vi "PTP.vi"() -> ()   [LabVIEW 2019]
panel:
  in  "Vision&Robot":T1(array[cluster])=[{"VisionPoint"={"X"=7.711431, "Y"=-4.299606}, "RobotPoint"={"X"=148.386, "Y"=76.831, "U"=0.0}}, {"VisionPoint"={"X"=213.378555, "Y"=-5.1972}, "RobotPoint"={"X"=351.958, "Y"=82.394, "U"=0.0}}, {"VisionPoint"={"X"=7.918081, "Y"=146.750031}, "RobotPoint"={"X"=152.021, "Y"=-78.481, "U"=0.0}}, {"VisionPoint"={"X"=220.545044, "Y"=146.174713}, "RobotPoint"={"X"=356.701, "Y"=-69.132, "U"=0.0}}, {"VisionPoint"={"X"=0.0, "Y"=0.0}, "RobotPoint"={"X"=0.0, "Y"=0.0, "U"=0.0}}, {"VisionPoint"={"X"=0.0, "Y"=0.0}, "RobotPoint"={"X"=0.0, "Y"=0.0, "U"=0.0}}, {"VisionPoint"={"X"=0.0, "Y"=0.0}, "RobotPoint"={"X"=0.0, "Y"=0.0, "U"=0.0}}]
  out "RobotOut(B )":cluster{"RX":dbl, "RY":dbl}
  in  "InputRobot(B)":T2
  in  "ImgPoint":T2
  in  "ImgPoint":cluster{"PTX1":dbl, "PTY1":dbl}
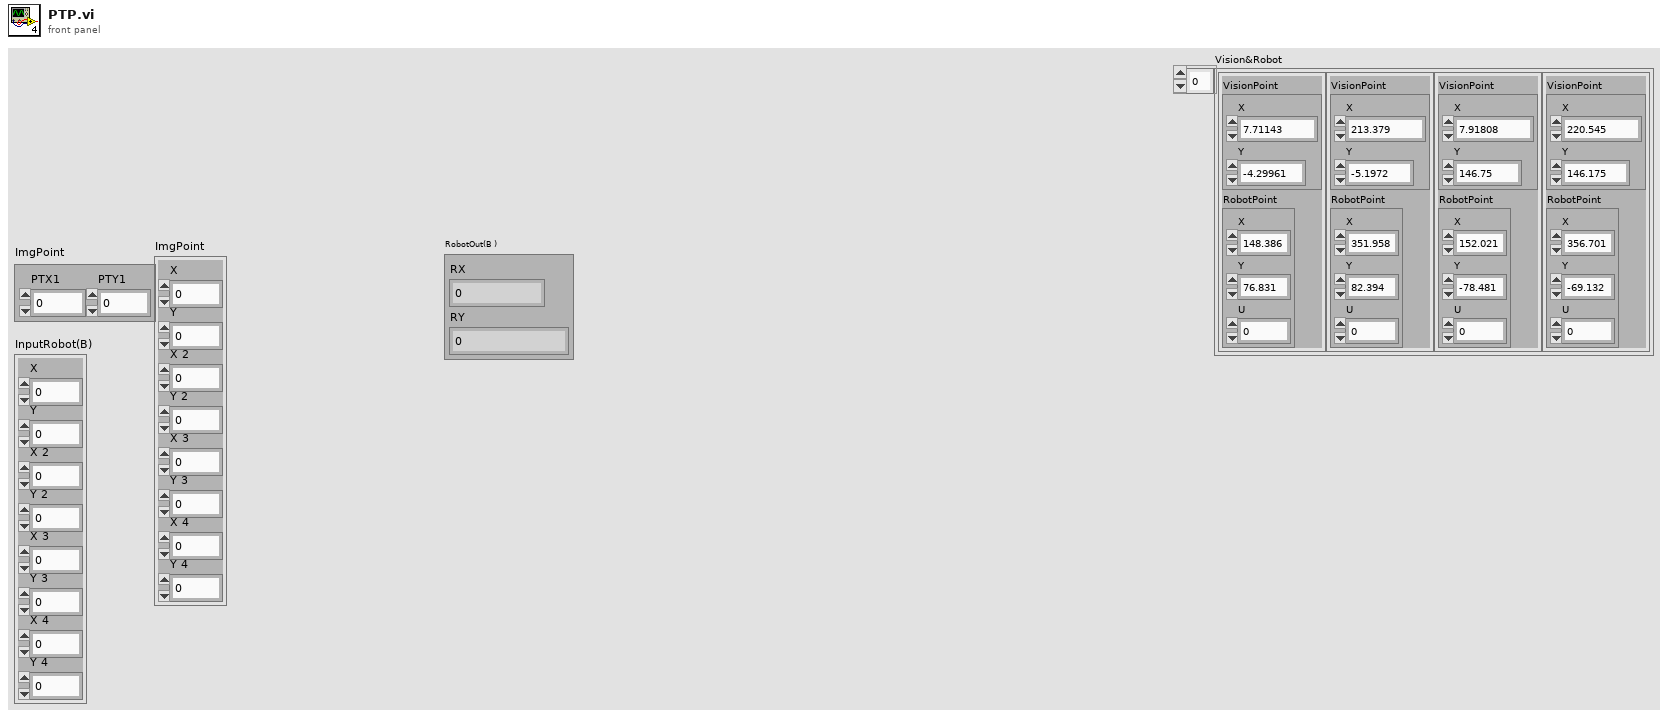
[diagram p1: front panel]
types:
  T1 = cluster{"VisionPoint":cluster{"X":dbl, "Y":dbl}, "RobotPoint":cluster{"X":dbl, "Y":dbl, "U":dbl}}[]
  T2 = cluster{"X":dbl, "Y":dbl, "X 2":dbl, "Y 2":dbl, "X 3":dbl, "Y 3":dbl, "X 4":dbl, "Y 4":dbl}
  T3 = cluster{"[0]":dbl, "[1]":dbl, "[2]":dbl, "[3]":dbl, "[4]":dbl, "[5]":dbl, "[6]":dbl, "[7]":dbl}
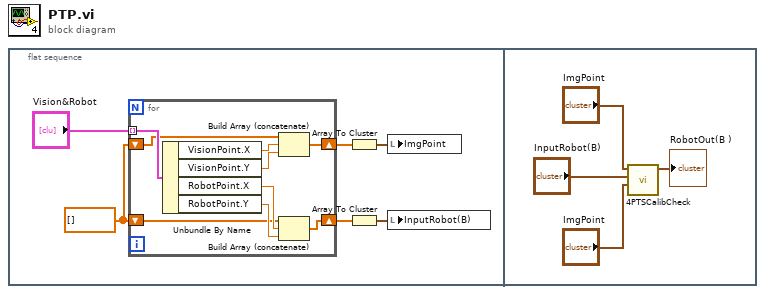
[diagram p0: block diagram]
diagram:
  n1 = flat-sequence {
    frame #0 {
      w3 = dbl[] []
      n2 = for {
        tunnel: "Vision&Robot" -> [w15] mode=indexing
        shift-right: [w12] -> w5
        shift-left: w3 -> [w11]
        shift-right: [w8] -> w2
        shift-left: w3 -> [w7]
        n3 = Unbundle By Name(w15) -> ("VisionPoint.X"=w9:dbl, "VisionPoint.Y"=w10:dbl, "RobotPoint.X"=w14:dbl, "RobotPoint.Y"=w13:dbl)
        n4 = Build Array (concatenate)(w7, w9, w10) -> (w8:dbl[])
        n5 = Build Array (concatenate)(w11, w14, w13) -> (w12:dbl[])
      }
      n6 = Array To Cluster(array=w2) -> (cluster=w1:T3)
      n7 = Array To Cluster(array=w5) -> (cluster=w4:T3)
      n8 = local write "ImgPoint"(w1) -> ()
      n9 = local write "InputRobot(B)"(w4) -> ()
    }
    frame #1 {
      n10 = call "4PTSCalibCheck.vi"("IdealPointIn(A)"="ImgPoint", "InputRobot(B)"="InputRobot(B)", "InputIdeal(A)"="ImgPoint") -> ("RobotOut(B )"=→"RobotOut(B )":cluster{"RX":dbl, "RY":dbl})  [unwired: 8 in]
    }
  }
